vi "OverlayBitmap.vi"() -> ()   [LabVIEW 2010]
panel:
  in  "stop":bool
  in  "ICImagingControl":refnum<k7>(container)
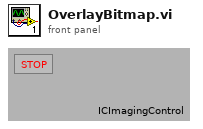
[diagram p1: front panel]
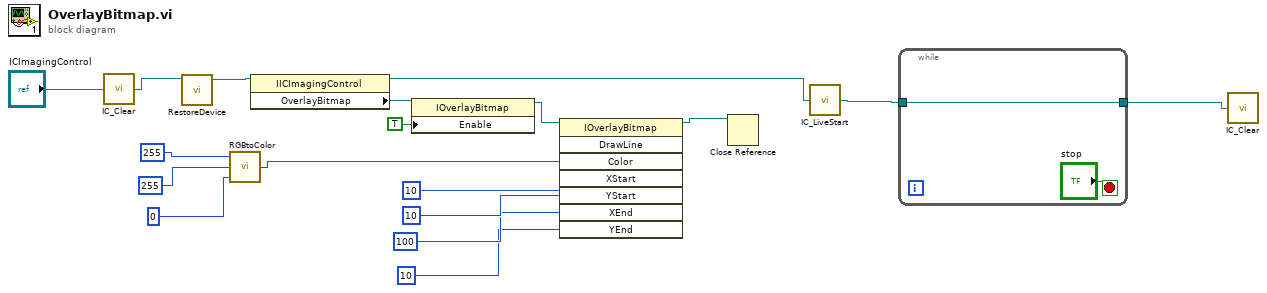
[diagram p0: block diagram]
diagram:
  n1 = call <userlib>:"IC_Clear.vi"("ICImagingControl 2"="ICImagingControl") -> ("ICImagingControl"=w17:refnum<k7>)
  n2 = call <userlib>:"RestoreDevice.vi"("ICImagingControl"=w17) -> ("ICImagingControl 2"=w14:refnum<k7>)  [unwired: 3 in, 2 out]
  n3 = call "RGBtoColor.vi"("Blue"=0 ("XStart"), "Green"=255 ("XStart"), "Red"=255 ("XStart")) -> ("Color"=w1:i32)
  n4 = property class="IICImagingControl"(reference=w14) -> (reference out=w6:refnum<k7>, "OverlayBitmap"=w13:refnum<k7>)  [unwired: 1 in, 1 out]
  n5 = property class="IOverlayBitmap"(reference=w13, "Enable"=TRUE) -> (reference out=w11:refnum<k7>)  [unwired: 1 in, 1 out]
  n6 = invoke class="IOverlayBitmap" method="DrawLine"(reference=w11, "Color"=w1, "XStart"=10, "YStart"=10, "XEnd"=100, "YEnd"=10) -> (reference out=w5:refnum<k7>)  [unwired: 2 in, 7 out]
  n7 = Close Reference(reference=w5) -> ()  [unwired: 1 in, 1 out]
  n8 = call <userlib>:"IC_LiveStart.vi"("ICImagingControl 3"=w6) -> ("ICImagingControl 2"=w16:refnum<k7>)
  n9 = while {
    tunnel: w16 -> [w19]
    tunnel: [w19] -> w15
    stop <- "stop" stop-if-true
  }
  n10 = call <userlib>:"IC_Clear.vi"("ICImagingControl 2"=w15) -> ()  [unwired: 1 out]
